vi "spec_ParseGratingSelectedString.vi"(8 "error in (no error)":errorcluster, 10 "GratingsSelected":string[](array[string]), 11 "LightField Automation in":refnum<class "LightField Automation.lvclass">) -> (0 "error out":errorcluster, 2 "Strings and Values Array":T1(array[cluster]), 3 "LightField Automation out":refnum<class "LightField Automation.lvclass">)   [LabVIEW 2018, in "LightField Automation.lvclass"]
uses:
  LightField Automation.lvclass
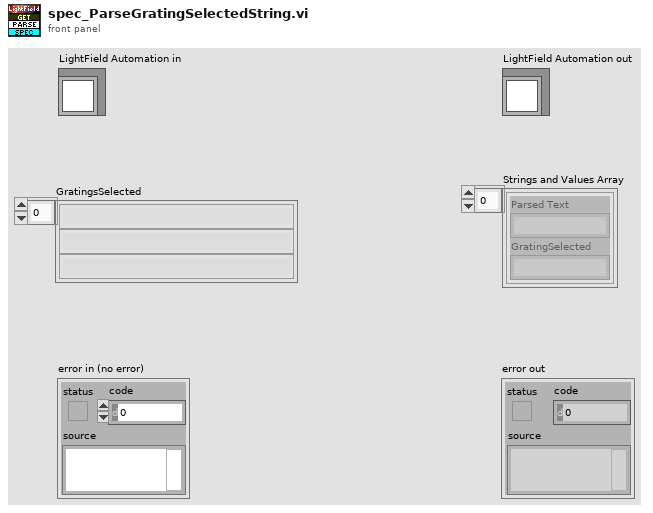
[diagram p1: front panel]
types:
  T1 = cluster{"Parsed Text":string, "GratingSelected":string}[]
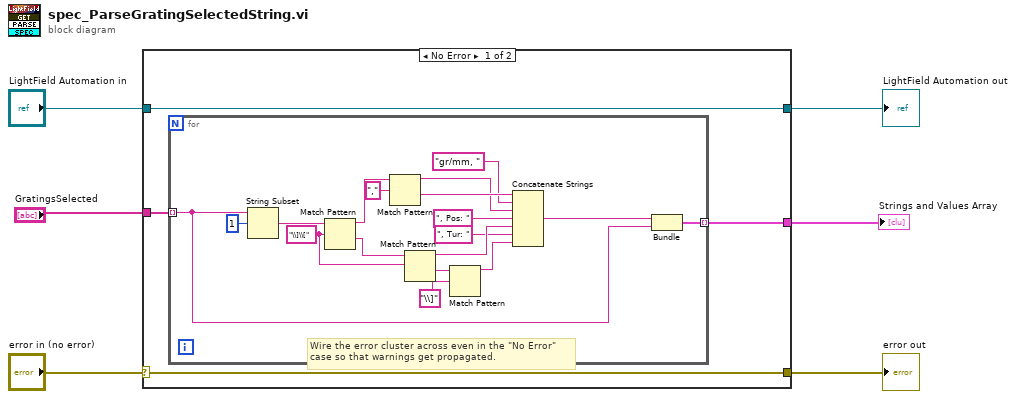
[diagram p0: block diagram]
diagram:
  n1 = case shown="No Error" "error in (no error)" {
    selector: "error in (no error)" -> [w9 w30]
    tunnel: [w9 w30] -> w5
    tunnel: [w10 w29] -> w3
    tunnel: "LightField Automation in" -> [w10 w29]
    tunnel: "GratingsSelected" -> [w8 _]
    tunnel: [w7 _] -> w1
    frame No Error {
      # "Wire the error cluster across even in the \"No Error\"\ncase so that warnings get propagated."
      n2 = for {
        tunnel: w8 -> [w12] mode=indexing
        tunnel: [w11] -> w7 mode=indexing
        w14 = "\\]\\[" ("regular expression")
        n3 = String Subset(string=w12, offset (0)=1) -> (substring=w27:string)  [unwired: 1 in]
        n4 = Match Pattern(string=w27, regular expression=w14) -> (before substring=w26:string, after substring=w24:string)  [unwired: 1 in, 2 out]
        n5 = Match Pattern(string=w26, regular expression=",") -> (before substring=w19:string, after substring=w21:string)  [unwired: 1 in, 2 out]
        n6 = Match Pattern(string=w24, regular expression=w14) -> (before substring=w17:string, after substring=w23:string)  [unwired: 1 in, 2 out]
        n7 = Match Pattern(string=w23, regular expression="\\]") -> (before substring=w15:string)  [unwired: 1 in, 3 out]
        n8 = Concatenate Strings(w21, "gr/mm, ", w19, ", Pos: " ("string"), w17, ", Tur: " ("string"), w15) -> (w13:string)
        n9 = Bundle(w13, "GratingSelected"=w12) -> (w11:cluster{string, "GratingSelected":string})  [unwired: 1 in]
      }
    }
    frame Error {
    }
  }
  "error out" <- w5
  "LightField Automation out" <- w3
  "Strings and Values Array" <- w1
